vi "MotionProfiles_NewPoints.vi"(8 "error in (no error)":errorcluster, 10 "CSV File Path":path=path "/home/lvuser/mp.csv", 11 "MotionProfiles in":refnum<class "MotionProfiles.lvclass">) -> (0 "error out":errorcluster, 3 "MotionProfiles out":refnum<class "MotionProfiles.lvclass">)   [LabVIEW 2016, in "MotionProfiles.lvclass"]
uses:
  MotionProfiles.lvclass
  <vilib>/Rock Robotics/WPI/ThirdParty/CanMotor/TalonSRX/WPI_CANTalonSRX_MotionProfileTrajectoryPt.ctl
  MotionProfiles.lvclass/MotionProfiles.ctl
  <vilib>/Utility/file.llb/Read Delimited Spreadsheet (DBL).vi
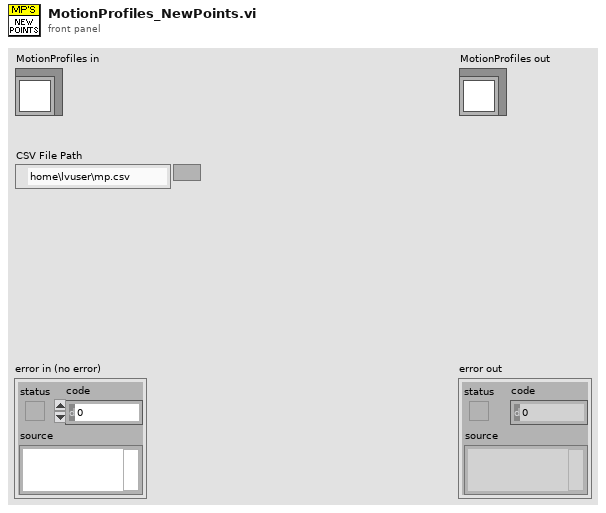
[diagram p1: front panel]
types:
  T1 = typedef "WPI_CANTalonSRX_MotionProfileTrajectoryPt.ctl" = cluster{"Duration Ms":u8, "Velocity":dbl, "Position":dbl, "Profile Slot Select":u8, "Is Last":bool, "Velocity Only":bool, "Zero Position":bool, "Compress Code":u8, "Same Velocity":i32, "Delta Position":i32, "Count":u8}
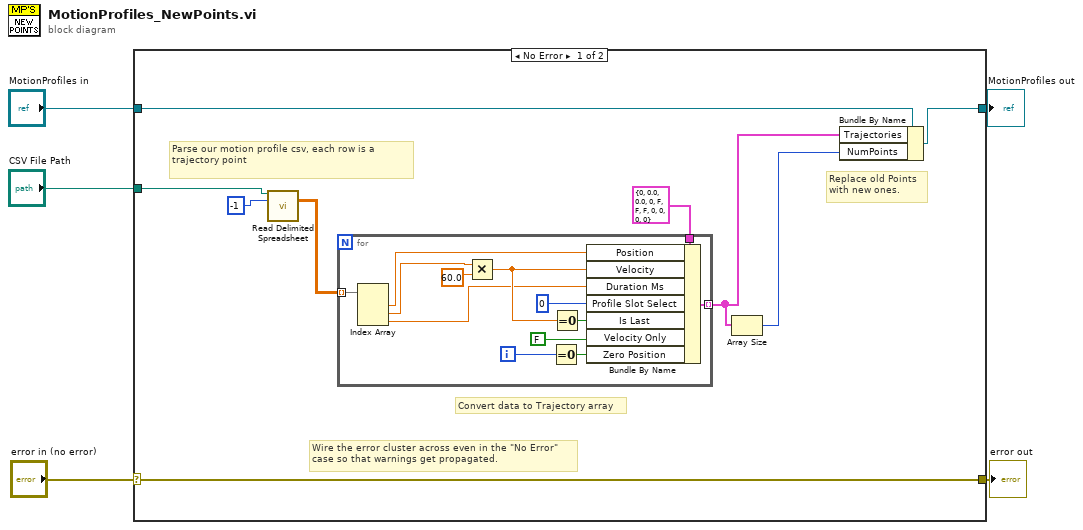
[diagram p0: block diagram]
diagram:
  n1 = case shown="No Error" "error in (no error)" {
    selector: "error in (no error)" -> [w14 w29]
    tunnel: [w14 w29] -> w4
    tunnel: [w10 w28] -> w2
    tunnel: "MotionProfiles in" -> [w11 w28]
    tunnel: "CSV File Path" -> [w12 _]
    frame No Error {
      # "Replace old Points\nwith new ones."
      # "Convert data to Trajectory array"
      # "Parse our motion profile csv, each row is a trajectory point"
      # "Wire the error cluster across even in the \"No Error\"\ncase so that warnings get propagated."
      n2 = call-poly <vilib>:"Read Delimited Spreadsheet.vi"("file path (dialog if empty)"=w12, "number of rows (all:-1)"=-1) -> ("all rows"=w6:dbl[][])  [unwired: 8 in, 5 out]
      n3 = for {
        tunnel: [w24] -> w8 mode=indexing
        tunnel: T1 {"Duration Ms"=0, "Velocity"=0.0, "Position"=0.0, "Profile Slot Select"=0, "Is Last"=FALSE, "Velocity Only"=FALSE, "Zero Position"=FALSE, "Compress Code"=0, "Same Velocity"=0, "Delta Position"=0, "Count"=0} -> [w19]
        tunnel: w6 -> [w18] mode=indexing
        i -> [w23]
        n4 = Index Array(array=w18) -> (element #1=w17:dbl, element #2=w16:dbl, element #3=w15:dbl)  [unwired: 3 in]
        n5 = Multiply(x=w16, y=60.0) -> (x*y=w21:dbl)
        n6 = Equal To 0?(x=w23) -> (x = 0?=w25:bool)
        n7 = Equal To 0?(x=w21) -> (x = 0?=w26:bool)
        n8 = Bundle By Name(cluster=w19, "Position"=w17, "Velocity"=w21, "Duration Ms"=w15, "Profile Slot Select"=u8 0, "Is Last"=w26, "Velocity Only"=FALSE, "Zero Position"=w25) -> (w24:T1)
      }
      n9 = Array Size(array=w8) -> (size(s)=w7:i32)
      n10 = Bundle By Name(cluster=w11, "Trajectories"=w8, "NumPoints"=w7) -> (w10:refnum<class "MotionProfiles.lvclass">)
    }
    frame Error {
    }
  }
  "error out" <- w4
  "MotionProfiles out" <- w2
